vi "even or odds.vi"(10 "x":dbl, 11 "x 2":dbl) -> (3 "f":dbl)   [LabVIEW 2014]
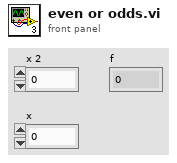
[diagram p1: front panel]
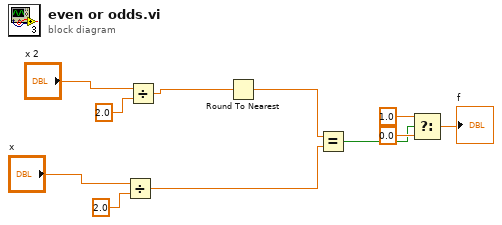
[diagram p0: block diagram]
diagram:
  n1 = Divide(x="x", y=2.0) -> (x/y=w7:dbl)
  n2 = Divide(x="x 2", y=2.0) -> (x/y=w5:dbl)
  n3 = Round To Nearest(number=w5) -> (nearest integer value=w6:dbl)
  n4 = Equal?(x=w6, y=w7) -> (x = y?=w8:bool)
  n5 = Select(t=1.0, s=w8, f=0.0) -> (s? t:f=→"f":dbl)
